vi "APRSOpen.vi"(6 "callsign for filter":string, 7 "filter?":bool=TRUE, 8 "Password":string, 9 "Login":string, 10 "port":dbl, 11 "server":string) -> (0 "error IO":errorcluster, 3 "conRef":T1)   [LabVIEW 2012]
doc: "This VI opens up a reference to a server and filters out the data you want."
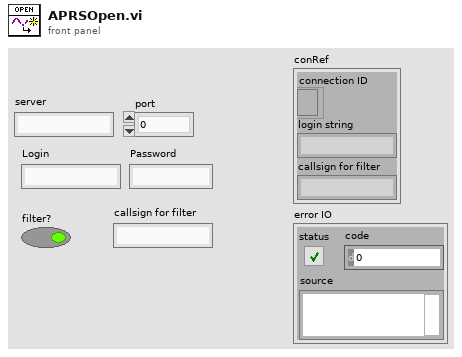
[diagram p1: front panel]
types:
  T1 = cluster{"connection ID":refnum<k5>, "login string":string, "callsign for filter":string}
  T2 = enum16{"Standard", "Buffered", "CRLF", "Immediate"}
  T3 = cluster{"connection ID":refnum<k5>, string, "callsign for filter":string}
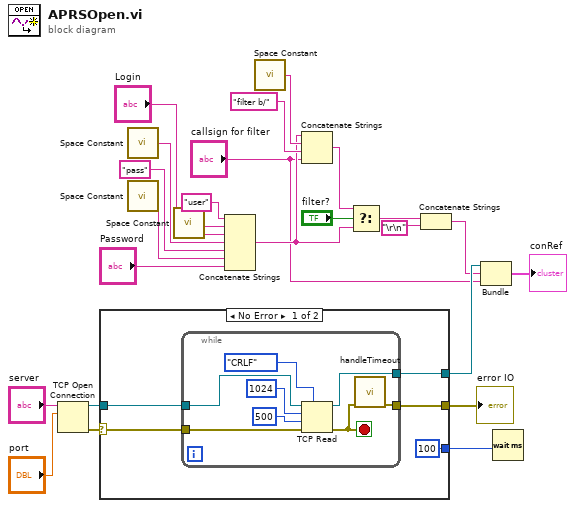
[diagram p0: block diagram]
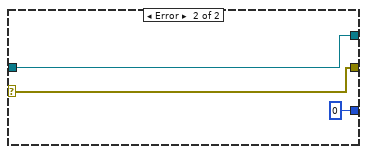
[diagram p2: hidden frame]
diagram:
  n1 = TCP Open Connection(address="server", remote port or service name="port") -> (connection ID=w22:refnum<k5>, error out=w23:errorcluster)  [unwired: 3 in]
  n2 = case shown="No Error" w23 {
    selector: w23 -> [w28 w40]
    tunnel: w22 -> [w29 w39]
    tunnel: [w26 w40] -> w20
    tunnel: [w27 w39] -> w5
    tunnel: [100 0] -> w1
    frame No Error {
      n3 = while {
        tunnel: w29 -> [w37]
        tunnel: [w36] -> w27
        tunnel: w28 -> [w35]
        tunnel: [w30] -> w26
        stop <- w31 stop-if-true
        n4 = TCP Read(connection ID=w37, bytes to read=1024, error in (no error)=w35, 7:T2."CRLF" ("mode (standard)"), 9:500 ("timeout ms (25000)")) -> (connection ID out=w36:refnum<k5>, error out=w31:errorcluster)  [unwired: 1 out]
        n5 = call "handleTimeout.vi"("error in (no error)"=w31) -> ("error out"=w30:errorcluster)  [unwired: 10 in]
      }
    }
    frame Error {
    }
  }
  "error IO" <- w20
  n6 = call <vilib>:"Space Constant.vi"() -> ("String"=w13:string)
  n7 = call <vilib>:"Space Constant.vi"() -> ("String"=w12:string)
  n8 = call <vilib>:"Space Constant.vi"() -> ("String"=w15:string)
  n9 = Concatenate Strings("user", w15, "Login", w13, "pass" ("string"), w12, "Password") -> (w8:string)
  n10 = call <vilib>:"Space Constant.vi"() -> ("String"=w16:string)
  n11 = Concatenate Strings(w8, w16, "filter b/" ("string"), "callsign for filter") -> (w9:string)
  n12 = Select(t=w9, s="filter?", f=w8) -> (s? t:f=w7:string)
  n13 = Concatenate Strings(w7, "\r\n") -> (w4:string)
  n14 = Bundle("connection ID"=w5, w4, "callsign for filter"="callsign for filter") -> (→"conRef":T3)  [unwired: 1 in]
  n15 = Wait (ms)(milliseconds to wait=w1) -> ()  [unwired: 1 out]
